vi "Find Extrema.vi"(3 "peaks/valleys":enum32{"Peaks", "Valleys"}(ring), 4 "Order (1)":u32=1, 5 "Array":dbl[](array[numeric])) -> (0 "# Zero Crossings":i32, 1 "Amplitudes":dbl[](array[numeric]), 2 "Indicies":u32[](array[numeric]))   [LabVIEW 2013, in "Empirical Mode Decomposition.lvlib"]
uses:
  Empirical Mode Decomposition.lvlib
panel:
  out "Last Value":dbl
  out "Value":dbl
  out "t":dbl
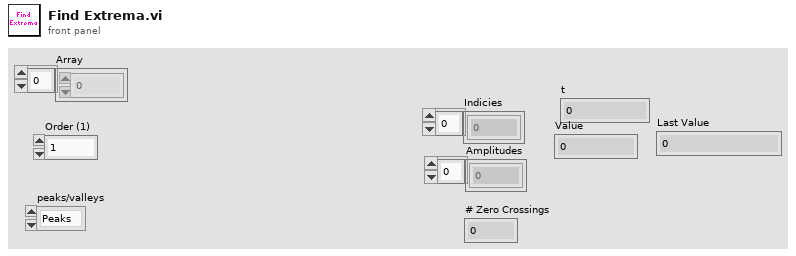
[diagram p1: front panel]
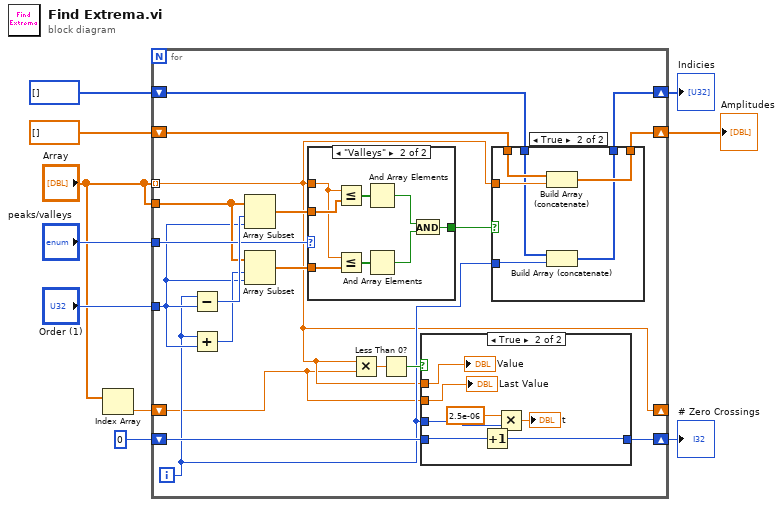
[diagram p0: block diagram]
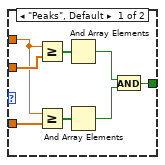
[diagram p4: hidden frame]
diagram:
  n1 = Index Array(array="Array") -> (element=w3:dbl)  [unwired: 1 in]
  n2 = for {
    tunnel: "Array" -> [w12] mode=indexing
    tunnel: "Order (1)" -> [w24]
    tunnel: "peaks/valleys" -> [w28]
    tunnel: "Array" -> [w26]
    shift-right: [w19] -> w5
    shift-left: dbl[] [] -> [w21]
    shift-right: [w18] -> w6
    shift-left: u32[] [] -> [w20]
    shift-right: [w12] -> _
    shift-left: w3 -> [w11]
    shift-right: [w14] -> w1
    shift-left: 0 -> [w15]
    i -> [w13]
    n3 = Subtract(x=w13, y=w24) -> (x-y=w29:u32)
    n4 = Add(x=w13, y=w24) -> (x+y=w25:u32)
    n5 = Array Subset(array=w26, index=w29, length=w24) -> (w27:dbl[])
    n6 = Array Subset(array=w26, index=w25, length=w24) -> (w23:dbl[])
    n7 = case shown="\"Valleys\"" w28 {
      tunnel: w27 -> [w53 w61]
      tunnel: w12 -> [w51 w59]
      tunnel: w23 -> [w52 w60]
      tunnel: [w46 w54] -> w22
      frame "Peaks", Default {
        n8 = Greater Or Equal?(x=w51, y=w53) -> (x >= y?=w50:bool[])
        n9 = Greater Or Equal?(x=w51, y=w52) -> (x >= y?=w49:bool[])
        n10 = And Array Elements(Boolean array=w50) -> (logical AND=w48:bool)
        n11 = And Array Elements(Boolean array=w49) -> (logical AND=w47:bool)
        n12 = And(x=w48, y=w47) -> (x .and. y?=w46:bool)
      }
      frame "Valleys" {
        n13 = Less Or Equal?(x=w59, y=w61) -> (x <= y?=w58:bool[])
        n14 = Less Or Equal?(x=w59, y=w60) -> (x <= y?=w57:bool[])
        n15 = And Array Elements(Boolean array=w58) -> (logical AND=w56:bool)
        n16 = And Array Elements(Boolean array=w57) -> (logical AND=w55:bool)
        n17 = And(x=w56, y=w55) -> (x .and. y?=w54:bool)
      }
    }
    n18 = Multiply(x=w12, y=w11) -> (x*y=w17:dbl)
    n19 = Less Than 0?(x=w17) -> (x < 0?=w16:bool)
    n20 = case shown="True" w16 {
      tunnel: w15 -> [w30 w37]
      tunnel: [w30 w36] -> w14
      tunnel: w13 -> [_ w33]
      tunnel: w12 -> [_ w35]
      tunnel: w11 -> [_ w34]
      frame False {
      }
      frame True {
        n21 = Increment(x=w37) -> (x+1=w36:i32)
        n22 = Multiply(x=2.5e-06, y=w33) -> (x*y=→"t":dbl)
        "Value" <- w35
        "Last Value" <- w34
      }
    }
    n23 = case shown="True" w22 {
      tunnel: w12 -> [_ w44]
      tunnel: w13 -> [_ w42]
      tunnel: w21 -> [w39 w45]
      tunnel: w20 -> [w38 w43]
      tunnel: [w39 w41] -> w19
      tunnel: [w38 w40] -> w18
      frame False {
      }
      frame True {
        n24 = Build Array (concatenate)(w45, w44) -> (w41:dbl[])
        n25 = Build Array (concatenate)(w43, w42) -> (w40:u32[])
      }
    }
  }
  "Indicies" <- w6
  "Amplitudes" <- w5
  "# Zero Crossings" <- w1
